vi "PH_Beckhoff_10BB_Plus.declare digital OutputTags.vi"(2 "Outputs to be inverted [#s separated by ::]":string, 3 "Instance Name":string="<Instance Name>") -> (0 "Digital Outputs":T2, 1 "Description":string)   [LabVIEW 2014, in "PH_Beckhoff_10BB_Plus.lvlib"]
uses:
  PH_Beckhoff_10BB_Plus.lvlib
  PH_Beckhoff/PH_Beckhoff.Digital Outputs.ctl
  PH_Beckhoff/PH_Beckhoff.lvlib
  PH_Beckhoff_Common/PH_Beckhoff_Common.lvlib
panel:
  in  "Digital Output Value":T1
  out "Right Size?":bool
  # "Let this VI run to check the size!"
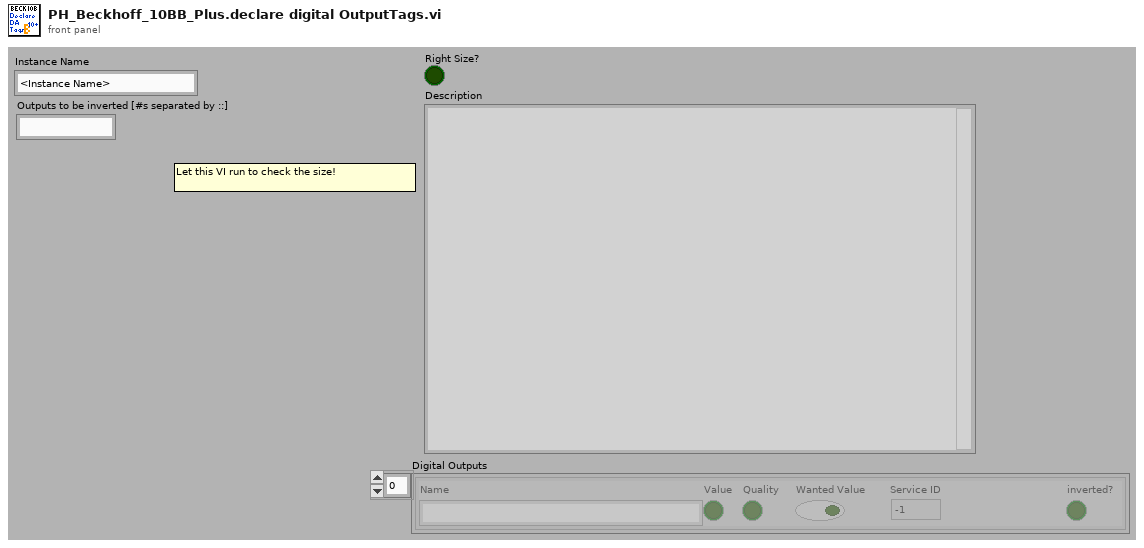
[diagram p1: front panel]
types:
  T1 = cluster{"Name":string, "Value":bool, "Quality":bool, "Wanted Value":bool, "Service ID":i32, "inverted?":bool}
  T2 = typedef "PH_Beckhoff.lvlib/PH_Beckhoff.Digital Outputs.ctl" = cluster{"Name":string, "Value":bool, "Quality":bool, "Wanted Value":bool, "Service ID":i32, "inverted?":bool}[]
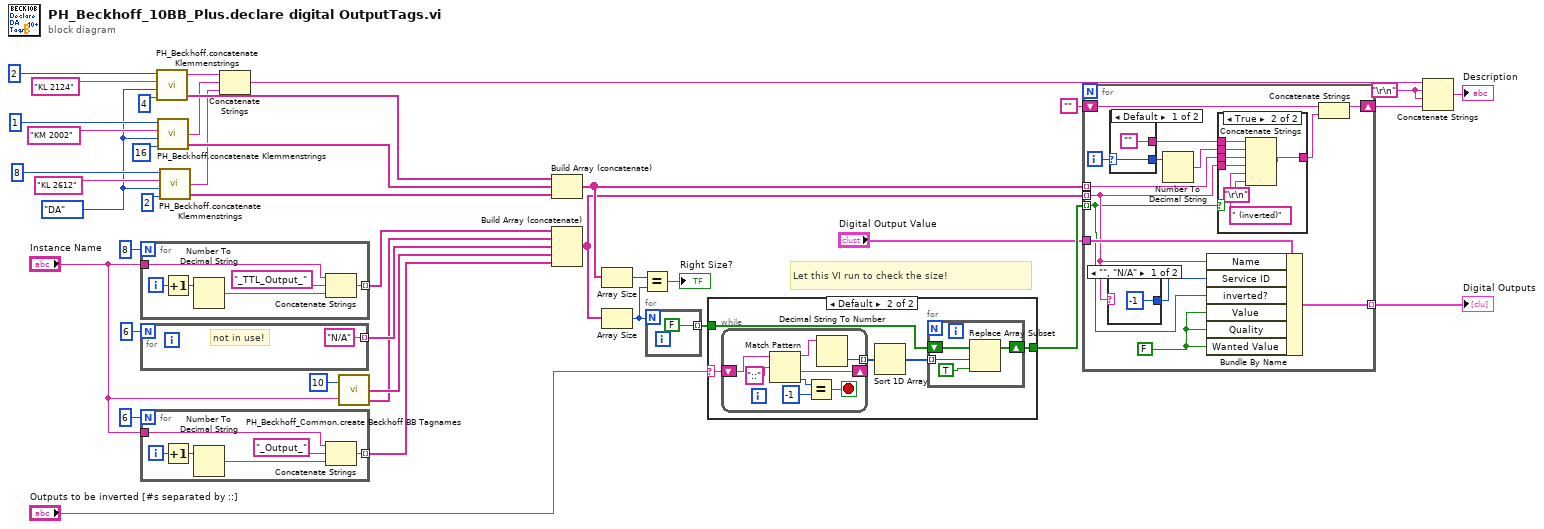
[diagram p0: block diagram]
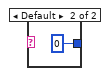
[diagram p2: hidden frame]
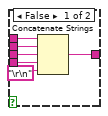
[diagram p3: hidden frame]
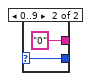
[diagram p4: hidden frame]
diagram:
  w40 = "\r\n"
  w23 = enum16{"AE", "AA", "DE", "DA"}."DA" ("Type")
  # "Let this VI run to check the size!"
  n1 = for {
    N: 8 -> [_]
    tunnel: [w43] -> w33 mode=indexing
    tunnel: "Instance Name" -> [w42]
    i -> [w47]
    n2 = Increment(x=w47) -> (x+1=w46:i32)
    n3 = Number To Decimal String(number=w46) -> (decimal integer string=w44:string)  [unwired: 1 in]
    n4 = Concatenate Strings(w42, "_TTL_Output_" ("string"), w44) -> (w43:string)
  }
  n5 = for {
    N: 6 -> [_]
    tunnel: ["N/A" ("string")] -> w30 mode=indexing
    # "not in use!"
  }
  n6 = for {
    N: 6 -> [_]
    tunnel: [w50] -> w32 mode=indexing
    tunnel: "Instance Name" -> [w49]
    i -> [w54]
    n7 = Increment(x=w54) -> (x+1=w53:i32)
    n8 = Number To Decimal String(number=w53) -> (decimal integer string=w51:string)  [unwired: 1 in]
    n9 = Concatenate Strings(w49, "_Output_" ("string"), w51) -> (w50:string)
  }
  n10 = call "PH_Beckhoff.concatenate Klemmenstrings.vi"("# of In- or Outputs"=4, "Type"=w23, "Klemmenname"="KL 2124", "Quantity"=2 ("size(s)")) -> ("concatenated string array"=w20:string[], "\"<Type>: <Quantity> x <Klemmenname>\""=w19:string)  [unwired: 1 out]
  n11 = call "PH_Beckhoff.concatenate Klemmenstrings.vi"("# of In- or Outputs"=16, "Type"=w23, "Klemmenname"="KM 2002", "Quantity"=1 ("size(s)")) -> ("concatenated string array"=w21:string[], "\"and <Quantity> x <Klemmenname>\""=w18:string)  [unwired: 1 out]
  n12 = call "PH_Beckhoff.concatenate Klemmenstrings.vi"("# of In- or Outputs"=2, "Type"=w23, "Klemmenname"="KL 2612", "Quantity"=8 ("size(s)")) -> ("concatenated string array"=w22:string[], "\"and <Quantity> x <Klemmenname>\""=w17:string)  [unwired: 1 out]
  n13 = Concatenate Strings(w19, w18, w17) -> (w16:string)
  n14 = call "PH_Beckhoff_Common.create Beckhoff BB Tagnames.vi"("#"=10, "Instance Name"="Instance Name") -> ("move-in-Tags"=w8:string[], "move-Tags"=w7:string[])  [unwired: 1 out]
  n15 = Build Array (concatenate)(w20, w21, w22) -> (w12:string[])
  n16 = Build Array (concatenate)(w33, w7, w30, w8, w32) -> (w3:string[])
  n17 = Array Size(array=w12) -> (size(s)=w36:i32)
  n18 = Array Size(array=w3) -> (size(s)=w6:i32)
  n19 = Equal?(x=w36, y=w6) -> (x = y?=→"Right Size?":bool)
  n20 = for {
    N: w6 -> [_]
    tunnel: [FALSE] -> w15 mode=indexing
  }
  n21 = case shown="Default" "Outputs to be inverted [#s separated by ::]" {
    selector: "Outputs to be inverted [#s separated by ::]" -> [_ w61]
    tunnel: w15 -> [w56 w58]
    tunnel: [w56 w57] -> w5
    frame "", "N/A" {
    }
    frame Default {
      n22 = while {
        shift-right: [w68] -> _
        shift-left: w61 -> [w73]
        tunnel: [w66] -> w60 mode=indexing
        stop <- w69 stop-if-true
        n23 = Match Pattern(string=w73, regular expression="::") -> (before substring=w67:string, after substring=w68:string, offset past match=w71:i32)  [unwired: 1 in, 1 out]
        n24 = Equal?(x=w71, y=-1) -> (x = y?=w69:bool)
        n25 = Decimal String To Number(string=w67) -> (number=w66:i32)  [unwired: 2 in, 1 out]
      }
      n26 = Sort 1D Array(array=w60) -> (sorted array=w59:i32[])
      n27 = for {
        tunnel: w59 -> [w63] mode=indexing
        shift-right: [w64] -> w57
        shift-left: w58 -> [w65]
        n28 = Replace Array Subset(array=w65, new element=TRUE ("new element/subarray"), index=w63) -> (w64:bool[])
      }
    }
  }
  n29 = for {
    tunnel: w3 -> [w78] mode=indexing
    tunnel: w12 -> [w83] mode=indexing
    shift-right: [w81] -> w11
    shift-left: "" -> [w80]
    tunnel: w5 -> [w76] mode=indexing
    tunnel: "Digital Output Value" -> [w79]
    tunnel: [w74] -> w1 mode=indexing
    i -> [w87]
    w75 = FALSE ("Quality")
    n30 = case shown="\"\", \"N/A\"" w78 {
      tunnel: [-1 0] -> w77
      frame "", "N/A" {
      }
      frame Default {
      }
    }
    n31 = case shown="Default" w87 {
      selector: w87 -> [w103 w106]
      tunnel: [w103 w106] -> w86
      tunnel: ["" "0"] -> w85
      frame Default {
      }
      frame 0..9 {
      }
    }
    n32 = Number To Decimal String(number=w86) -> (decimal integer string=w84:string)  [unwired: 1 in]
    n33 = Bundle By Name(cluster=w79, "Name"=w78, "Service ID"=w77, "inverted?"=w76, "Value"=w75, "Quality"=w75, "Wanted Value"=w75) -> (w74:T1)
    n34 = case shown="True" w76 {
      tunnel: w85 -> [w95 w102]
      tunnel: w84 -> [w94 w101]
      tunnel: w83 -> [w93 w100]
      tunnel: w78 -> [w92 w99]
      tunnel: [w90 w97] -> w82
      frame False {
        n35 = Concatenate Strings(w95, w94, w93, w92, "\r\n") -> (w90:string)
      }
      frame True {
        n36 = Concatenate Strings(w102, w101, w100, w99, " (inverted)", "\r\n") -> (w97:string)
      }
    }
    n37 = Concatenate Strings(w80, w82) -> (w81:string)
  }
  "Digital Outputs" <- w1
  n38 = Concatenate Strings(w16, w40, w40, w11) -> (→"Description":string)
